vi "IV_curve_measurement.vi"(0 "Dwell Time (ms)":u32, 1 "V array in (V)":dbl[](array[numeric]), 2 "I array in (A)":dbl[](array[numeric]), 3 "Collected array in":dbl[][](array[numeric]), 4 "B array in (T)":dbl[](array[numeric]), 5 "Set V":dbl=0.3, 7 "dV":dbl, 9 "MaxV":dbl) -> (6 "Best Linear Fit":dbl[](array[numeric]), 8 "appended array":dbl[][](array[numeric]), 10 "I array out (pA)":dbl[](array[numeric]), 11 "Boolean":bool, 12 "V array out (V)":dbl[](array[numeric]), 13 "intercept 2":dbl, 14 "Collected array out":dbl[][](array[numeric]), 15 "Vout":dbl, 17 "slope 2":dbl)   [LabVIEW 2015]
uses:
  <vilib>/Analysis/NI_AALPro.lvlib
panel:
  out "concatenated string":string
  in  "error in (no error)":errorcluster
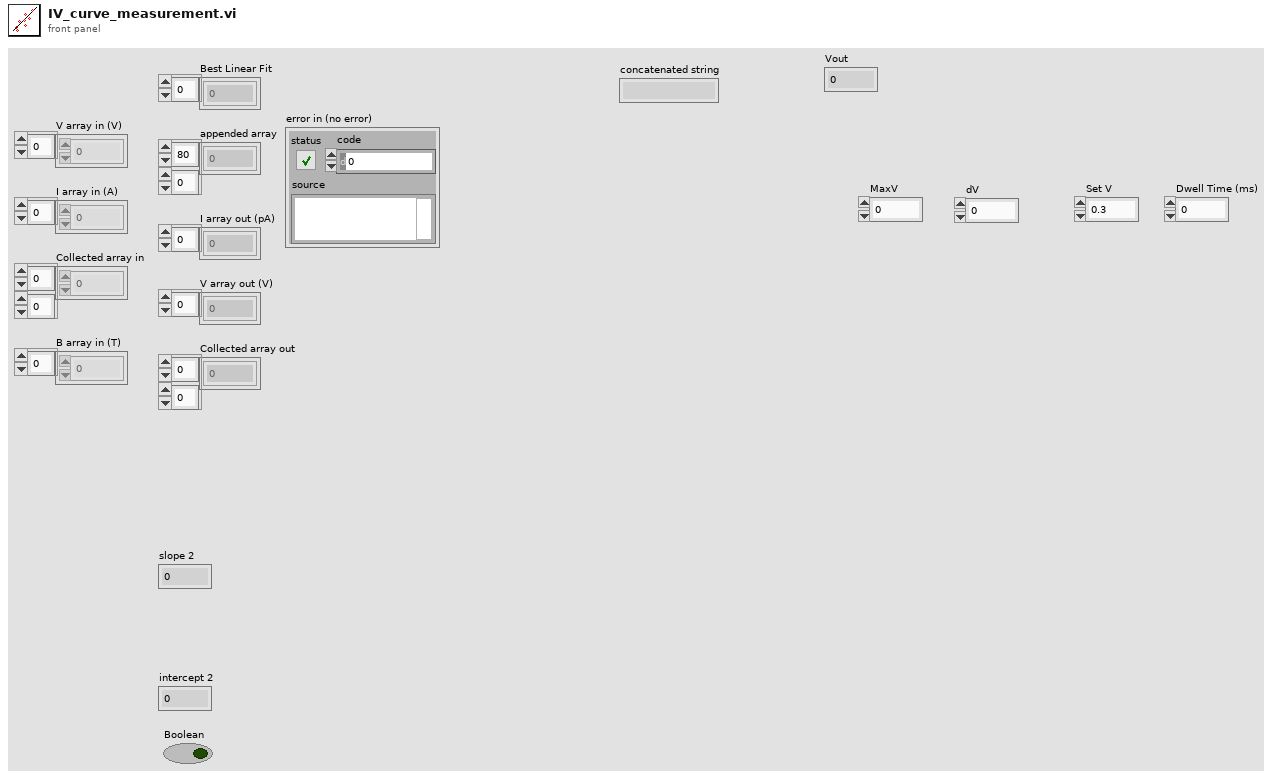
[diagram p1: front panel]
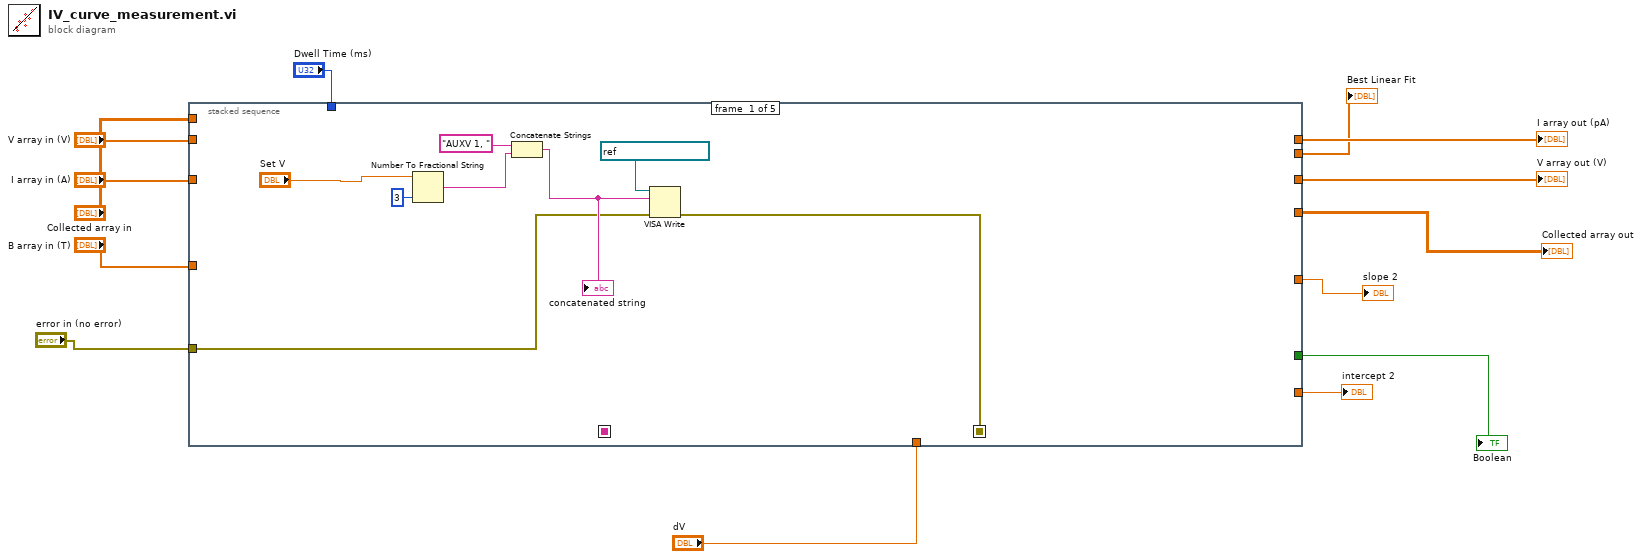
[diagram p0: block diagram]
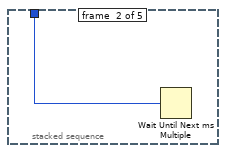
[diagram p2: hidden frame]
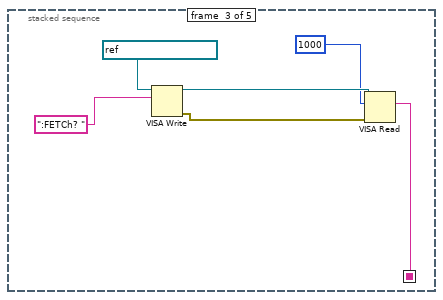
[diagram p3: hidden frame]
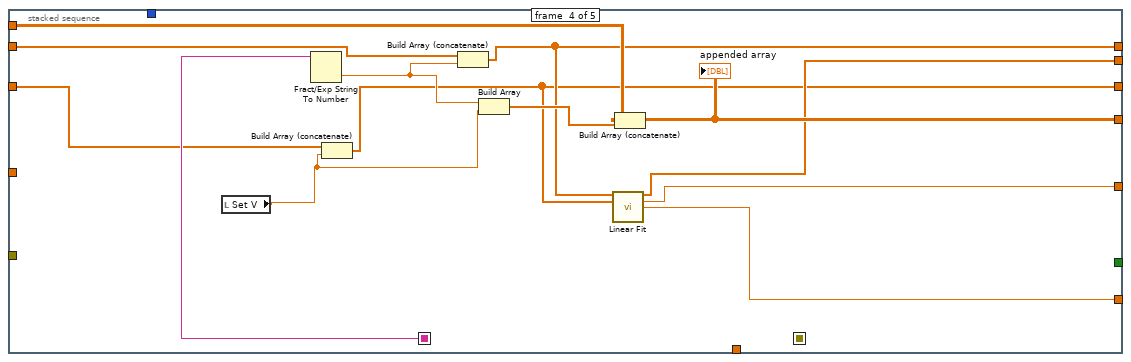
[diagram p4: hidden frame]
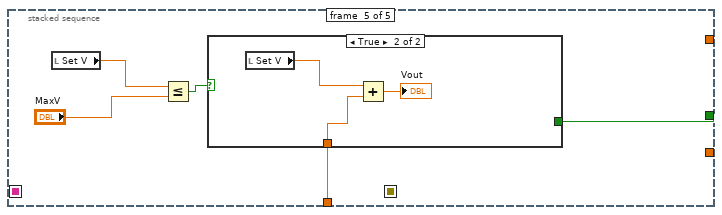
[diagram p5: hidden frame]
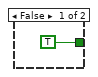
[diagram p6: hidden frame]
diagram:
  n1 = stacked-sequence {
    seq-local: [_ _ w24 _ _] -> [_ _ _ w39 _]
    seq-local: [w16 _ _ _ _] -> [_ _ _ _ _]
    tunnel: [_ _ _ w41 _] -> w2
    tunnel: "Collected array in" -> [_ _ _ w40 _]
    tunnel: [_ _ _ _ w46] -> w4
    tunnel: [_ _ _ w31 _] -> w9
    tunnel: "V array in (V)" -> [_ _ _ w38 _]
    tunnel: "B array in (T)" -> [_ _ _ _ _]
    tunnel: [_ _ _ w30 _] -> w10
    tunnel: "I array in (A)" -> [_ _ _ w37 _]
    tunnel: [_ _ _ w36 _] -> w8
    tunnel: [_ _ _ w34 _] -> w11
    tunnel: [_ _ _ w33 _] -> w12
    tunnel: "dV" -> [_ _ _ _ w45]
    tunnel: "Dwell Time (ms)" -> [_ w23 _ _ _]
    tunnel: "error in (no error)" -> [w17 _ _ _ _]
    frame #0 {
      n2 = Number To Fractional String(number="Set V", precision (6)=i16 3) -> (F-format string=w20:string)  [unwired: 2 in]
      n3 = Concatenate Strings("AUXV 1, " ("data"), w20) -> (w19:string)
      "concatenated string" <- w19
      n4 = VISA Write(VISA resource name=refnum<visa-resource-name> "GPIB0::5::INSTR", write buffer=w19, error in (no error)=w17) -> (error out=w16:errorcluster)  [unwired: 2 out]
    }
    frame #1 {
      n5 = Wait Until Next ms Multiple(millisecond multiple=w23) -> ()  [unwired: 1 out]
    }
    frame #2 {
      n6 = VISA Write(VISA resource name=refnum<visa-resource-name> "GPIB0::20::INSTR", write buffer=":FETCh? " ("data")) -> (VISA resource name out=w29:refnum<visa-resource-name>, error out=w25:errorcluster)  [unwired: 1 in, 1 out]
      n7 = VISA Read(VISA resource name=w29, byte count=u32 1000, error in (no error)=w25) -> (read buffer=w24:string)  [unwired: 3 out]
    }
    frame #3 {
      n8 = local read "Set V"() -> (w32:dbl)
      n9 = Fract/Exp String To Number(string=w39) -> (number=w35:dbl)  [unwired: 3 in, 1 out]
      n10 = Build Array (concatenate)(w37, w32) -> (w30:dbl[])
      n11 = Build Array (concatenate)(w38, w35) -> (w31:dbl[])
      n12 = Build Array(w35, w32) -> (w42:dbl[])
      n13 = call <vilib>:"Linear Fit.vi"("Y"=w31, "X"=w30) -> ("Best Linear Fit"=w36:dbl[], "slope"=w34:dbl, "intercept"=w33:dbl)  [unwired: 9 in, 2 out]
      n14 = Build Array (concatenate)(w40, w42) -> (w41:dbl[][])
      "appended array" <- w41
    }
    frame #4 {
      n15 = local read "Set V"() -> (w44:dbl)
      n16 = Less Or Equal?(x=w44, y="MaxV") -> (x <= y?=w47:bool)
      n17 = case shown="True" w47 {
        tunnel: [TRUE _] -> w46
        tunnel: w45 -> [_ w51]
        frame False {
        }
        frame True {
          n18 = local read "Set V"() -> (w50:dbl)
          n19 = Add(x=w50, y=w51) -> (x+y=→"Vout":dbl)
        }
      }
    }
  }
  "intercept 2" <- w12
  "slope 2" <- w11
  "V array out (V)" <- w10
  "I array out (pA)" <- w9
  "Best Linear Fit" <- w8
  "Boolean" <- w4
  "Collected array out" <- w2
